vi "Model - Get Elevator States.vi"(8 "error in (no error)":errorcluster, 11 "View Model":T2) -> (0 "error out":errorcluster, 1 "Elevator Next State":T1, 2 "Elevator State":T1, 3 "View Model":T2)   [LabVIEW 2017]
doc: "Get Elevator states values from View Model's DVR"
uses:
  Controls/View Model.ctl
  Configuration/Controls/Config Model.ctl
  Configuration/Controls/Config Data.ctl
  Error Handler/Controls/Error Model.ctl
  Error Handler/Controls/Error Data.ctl
  Error Handler/Controls/Error Type.ctl
  Controls/Shared Model.ctl
  Elevator Controller/Controls/Elevator Model.ctl
  Elevator Controller/Controls/Elevator Location.ctl
  Elevator Controller/Controls/Elevator CMD Data.ctl
  Elevator Controller/Controls/Elevator Commands.ctl
  Elevator Controller/Controls/Elevator Overhead.ctl
  Elevator Controller/Controls/Elevator States.ctl
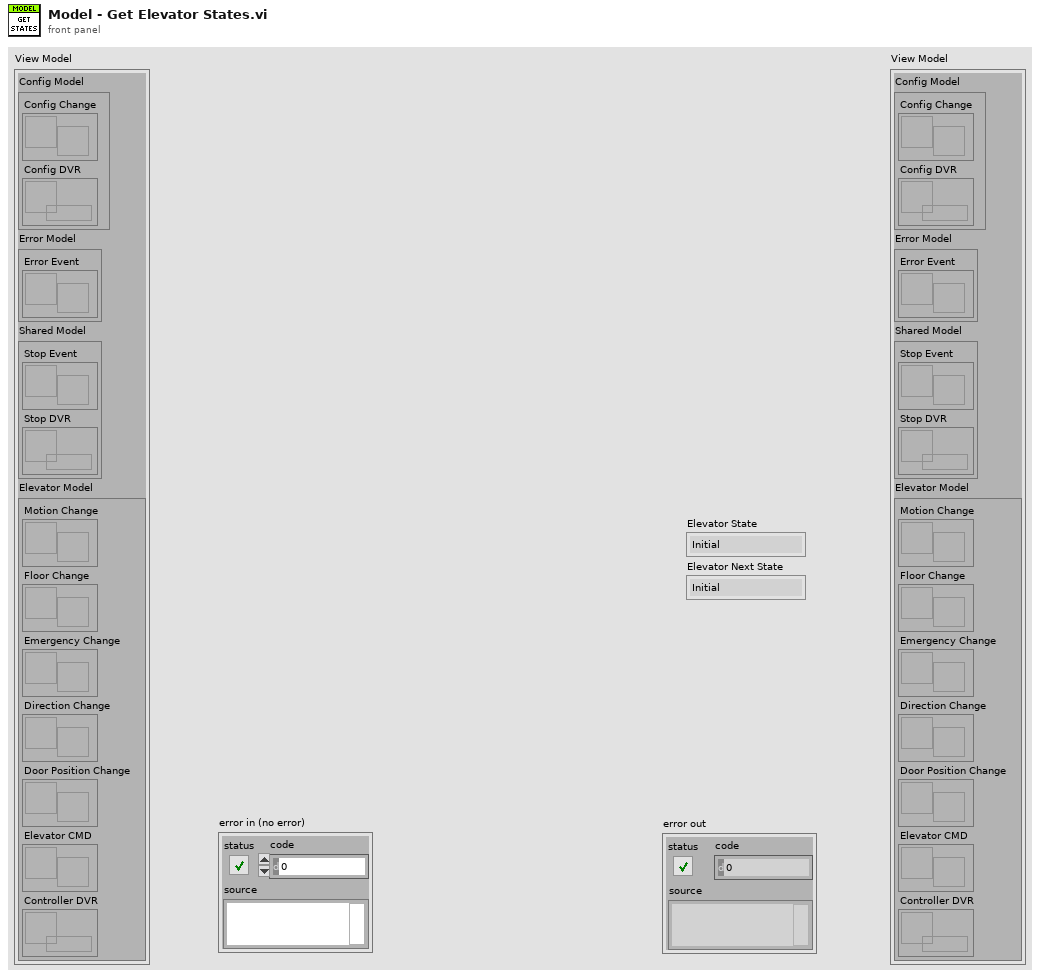
[diagram p1: front panel]
types:
  T1 = typedef "Elevator States.ctl" = enum16{"Initial", "Wait for 1st Request", "Start and Move", "Analysis", "Continue Travel", "Stop at Floor", "Open and Close Door", "No Request", "Emergency", "Terminate"}
  T2 = typedef "View Model.ctl" = cluster{"Config Model":T3, "Error Model":T4, "Shared Model":T5, "Elevator Model":T6}
  T3 = typedef "Config Model.ctl" = cluster{"Config Change":refnum<user-event>, "Config DVR":refnum<data-value>}
  T4 = typedef "Error Model.ctl" = cluster{"Error Event":refnum<user-event>}
  T5 = typedef "Shared Model.ctl" = cluster{"Stop Event":refnum<user-event>, "Stop DVR":refnum<data-value>}
  T6 = typedef "Elevator Model.ctl" = cluster{"Motion Change":refnum<user-event>, "Floor Change":refnum<user-event>, "Emergency Change":refnum<user-event>, "Direction Change":refnum<user-event>, "Door Position Change":refnum<user-event>, "Elevator CMD":refnum<user-event>, "Controller DVR":refnum<data-value>}
  T7 = typedef "Elevator Overhead.ctl" = cluster{"In Motion?":bool, "Direction":bool, "Door Movement":bool, "Door Position":bool, "Timer":dbl, "Elapsed Time":dbl, "Elevator State":T1, "Elevator Next State":T1}
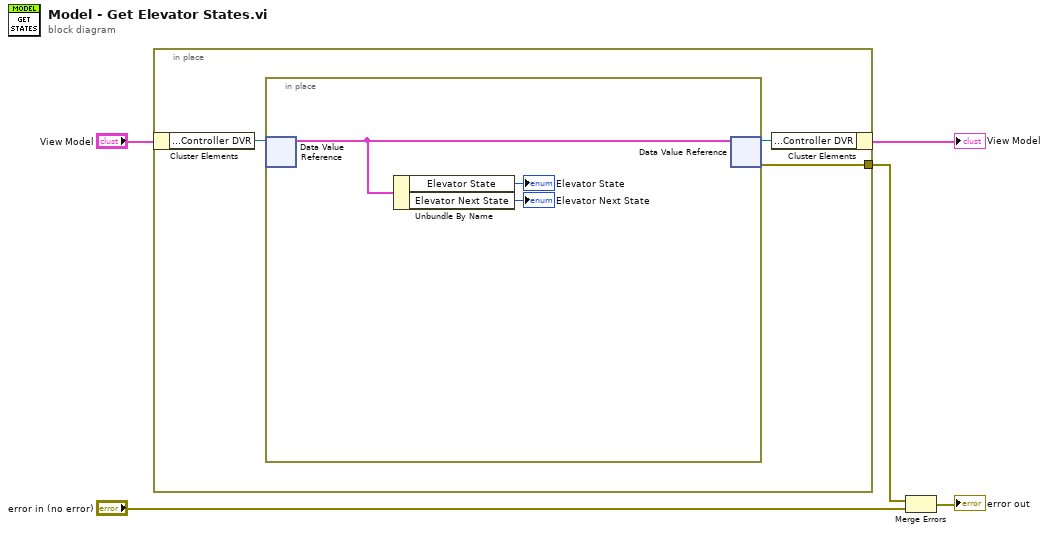
[diagram p0: block diagram]
diagram:
  n1 = in-place {
    in-place-border: [w6] -> w2
    n2 = in-place-cluster #1("View Model") -> ("Elevator Model.Controller DVR"=w8:refnum<data-value>)
    n3 = in-place {
      n4 = in-place-dvr #2(w8) -> (w11:T7)  [unwired: 1 out]
      n5 = Unbundle By Name(w11) -> ("Elevator State"=→"Elevator State":T1, "Elevator Next State"=→"Elevator Next State":T1)
      n6 = in-place-dvr #2(w11) -> (w7:refnum<data-value>, w6:errorcluster)
    }
    n7 = in-place-cluster #1("Elevator Model.Controller DVR"=w7) -> (→"View Model":T2)
  }
  n8 = Merge Errors(w2, "error in (no error)") -> (→"error out":errorcluster)
